vi "Kinesis-get-motor-ID.vi"() -> ()   [LabVIEW 2014]
doc: "André Romero - 2017\nandretec@ifsc.usp.br"
panel:
  in  "stop":bool
  out "GetPOS":dbl
  out "SerialNumber":u32
  out "Motor 1":bool
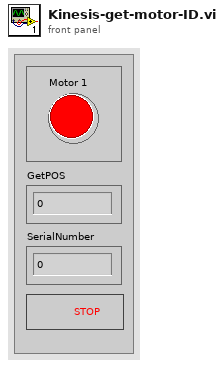
[diagram p1: front panel]
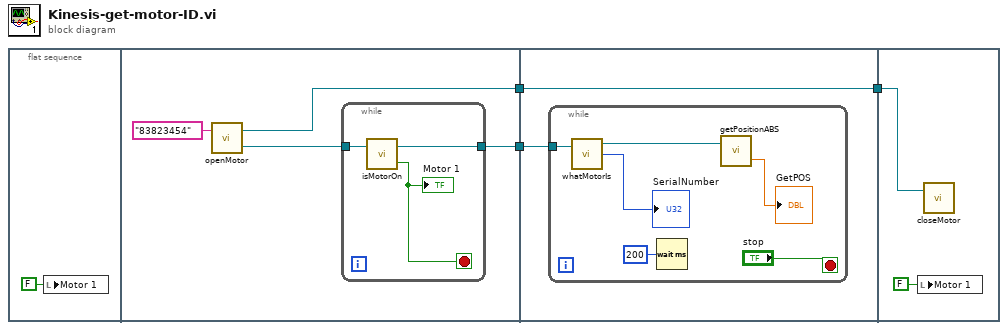
[diagram p0: block diagram]
diagram:
  n1 = flat-sequence {
    tunnel: [w8] -> w3
    tunnel: [w7] -> w2
    tunnel: w3 -> [w12]
    tunnel: [w13] -> w1
    tunnel: w2 -> [w13]
    tunnel: w1 -> [w21]
    frame #0 {
      n2 = local write "Motor 1"(FALSE ("Motor 1")) -> ()
    }
    frame #1 {
      n3 = call "openMotor.vi"("S/N Motor"="83823454") -> ("Device"=w6:refnum<k24>, ".NET Refnum out"=w7:refnum<k24>)  [unwired: 1 in]
      n4 = while {
        tunnel: w6 -> [w11]
        tunnel: [w10] -> w8
        stop <- w9 stop-if-true
        n5 = call "isMotorOn.vi"("Device"=w11) -> ("isConnected"=w9:bool, "Device out"=w10:refnum<k24>)  [unwired: 1 in]
        "Motor 1" <- w9
      }
    }
    frame #2 {
      n6 = while {
        tunnel: w12 -> [w16]
        stop <- "stop" stop-if-true
        n7 = call "whatMotorIs.vi"("Device in"=w16) -> ("SerialNumber"=→"SerialNumber":u32, "Device out"=w18:refnum<k24>)  [unwired: 3 in]
        n8 = Wait (ms)(milliseconds to wait=u32 200) -> ()  [unwired: 1 out]
        n9 = call "getPositionABS.vi"("Device"=w18) -> ("GetPOS"=→"GetPOS":dbl)  [unwired: 1 in, 1 out]
      }
    }
    frame #3 {
      n10 = local write "Motor 1"(FALSE ("Motor 1")) -> ()
      n11 = call "closeMotor.vi"(".NET Refnum in"=w21) -> ()  [unwired: 2 in]
    }
  }
